vi "__init__.vi"(8 "error in (no error)":errorcluster, 11 "SsaId in":refnum<class "SsaId.lvclass">) -> (0 "error out":errorcluster, 3 "SsaId out":refnum<class "SsaId.lvclass">)   [LabVIEW 2020, in "mlir.lvlib" / "SsaId.lvclass"]
uses:
  SsaId.lvclass
  SsaId.lvclass/SsaId.ctl
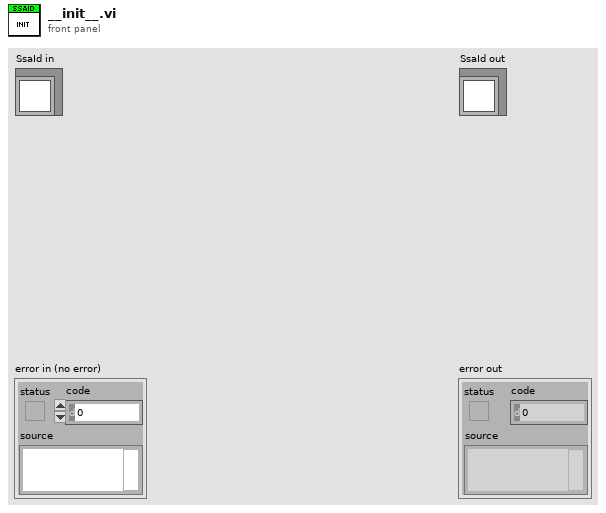
[diagram p1: front panel]
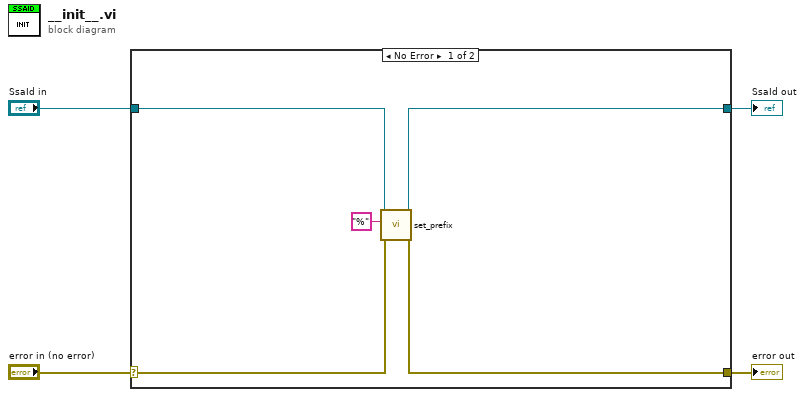
[diagram p0: block diagram]
diagram:
  n1 = case shown="No Error" "error in (no error)" {
    selector: "error in (no error)" -> [w6 w11]
    tunnel: [w5 w11] -> w3
    tunnel: [w9 w10] -> w1
    tunnel: "SsaId in" -> [w8 w10]
    frame No Error {
      n2 = call-dynamic "set_prefix.vi"("error in (no error)"=w6, "_prefix_"="%", "self in"=w8) -> ("error out"=w5:errorcluster, "self out"=w9:refnum<class "SsaId.lvclass">)  [unwired: 7 in]
    }
    frame Error {
    }
  }
  "error out" <- w3
  "SsaId out" <- w1
